vi "HEWH Check Cutout.vi"(0 "Station":string="A", 1 "Use Cutout Delay":bool, 3 "Debug":bool, 5 "Debug Events":T8, 7 "Station Data Input":T1={"Sequence #"=0.0, "Cycles"=0, "Mode Setting"="", "Flow Rate (GPM)"=0.0, "Temperature (F)"=0.0, "Reset Timer"=FALSE, "Use Temp Decline Method"=FALSE, "Terminate Condition"=enum."C1-Terminate Draw @ Gallon Mark", "Condition Value #1"=0.0, "UE"=FALSE, "LE"=FALSE, "Comp"=FALSE, "Fan"=FALSE, "Test End Time (Sec)"=0.0, "Purge Until Cutout"=FALSE, "Start Conditions"=enum."Heat Source Cutout", "Condition Value #2"=0.0, "Remove Power"=FALSE, "Time"=0.0, "Check Special Cond."=enum."SC2-Check Heat Source (On-C2/Off-C1)", "Condition#"=enum."C1", "Draw Flags"=enum."N/A", "Data Processing Delay (FHD 15sec, UEF 5 Sec)"=0.0, "Test Complete"=FALSE} {"Time" format="%<%H:%M:%S>t"}, 9 "Current (Amps)":dbl=1.0, 11 "Error In":errorcluster, 12 "Delay After Cutout (sec)":dbl=1.0, 14 "Start Draw":bool) -> (4 "Full Cutout?":bool, 15 "Error Out":errorcluster)   [LabVIEW 2016]
uses:
  Type Definitions/HEWH Power Elements.ctl
  Type Definitions/PRAT Test.ctl
  Utility/Save File/File Setup (Public)/Type Definition/Save File HEWH Heating Control Mode.ctl
  Draw Water Specific/Type Definitions/Terminate Draw Conditions.ctl
  Type Definitions/HEWH Start Conditions.ctl
  Draw Water Specific/Type Definitions/Check Special Condtions.ctl
  Draw Water Specific/Type Definitions/HEWH Special Condition Check.ctl
  Type Definitions/HEWH Draw Flag ENUM.ctl
  Utility/Type Definitions/UTILITY Notifier.ctl
  Utility/Save File/File Setup.lvlib
panel:
  out "Heat Source ON (1=ON)":bool
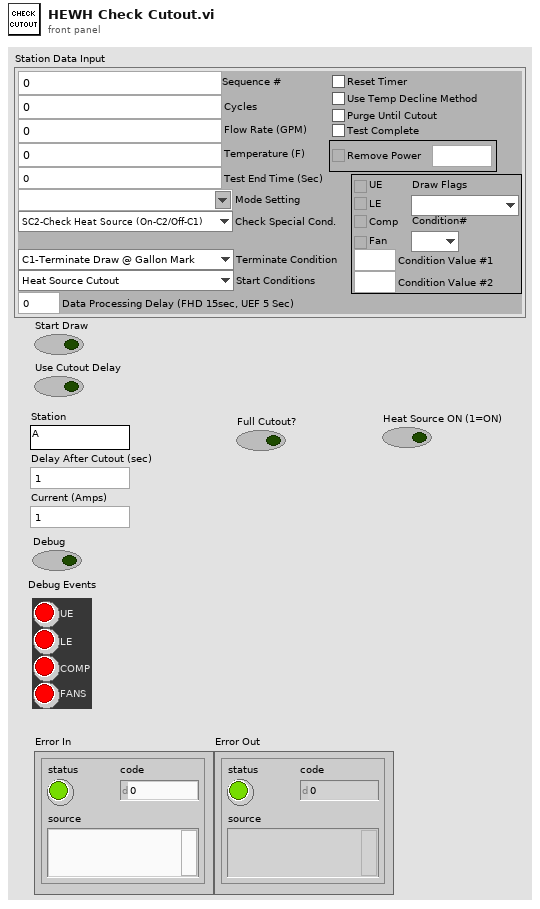
[diagram p1: front panel]
types:
  T1 = typedef "PRAT Test.ctl" = cluster{"Sequence #":dbl, "Cycles":i32, "Mode Setting":T2, "Flow Rate (GPM)":dbl, "Temperature (F)":dbl, "Reset Timer":bool, "Use Temp Decline Method":bool, "Terminate Condition":T3, "Condition Value #1":dbl, "UE":bool, "LE":bool, "Comp":bool, "Fan":bool, "Test End Time (Sec)":dbl, "Purge Until Cutout":bool, "Start Conditions":T4, "Condition Value #2":dbl, "Remove Power":bool, "Time":dbl, "Check Special Cond.":T5, "Condition#":T6, "Draw Flags":T7, "Data Processing Delay (FHD 15sec, UEF 5 Sec)":dbl, "Test Complete":bool}
  T2 = typedef "File Setup.lvlib/Save File HEWH Heating Control Mode.ctl" = string
  T3 = typedef "Terminate Draw Conditions.ctl" = enum16{"C1-Terminate Draw @ Gallon Mark", "C2-Special Last Draw (HU Test)", "C3-RTD Out <=", "C4-Mean Tank Temp <=", "C5-Decrease RTD Out (Deg F)", "C6-Time (Seconds)", "C7-Until Any Heat Source", "C8-Specific Heat Source", "C9-Do Nothing"}
  T4 = typedef "HEWH Start Conditions.ctl" = enum16{"Heat Source Cutout", "At Time (Seconds)", "Every X (Seconds)", "T2 >= X° Below Setpoint", "Seconds From Complete", "Wait for LE & Comp Cutout", "Wait for Comp Cutout", "Wait for LE Cutout", "Wait for UE Cutout"}
  T5 = typedef "Check Special Condtions.ctl" = enum16{"SC1-Do Nothing", "SC2-Check Heat Source (On-C2/Off-C1)", "SC3-Check Skip Condition", "SC4-Check Heat Source ON/Fail"}
  T6 = typedef "HEWH Special Condition Check.ctl" = enum16{"N/A", "C1", "C2", "Reset/Fail", "Skip Draw Sequence"}
  T7 = typedef "HEWH Draw Flag ENUM.ctl" = enum16{"N/A", "None(0)", "Sml(1)", "Med(2)", "SmlMed(3)", "Lrg(4)", "SmlLrg(5)", "MedLrg(6)", "SmlMedLrg(7)"}
  T8 = typedef "HEWH Power Elements.ctl" = cluster{"UE":bool, "LE":bool, "COMP":bool, "FANS":bool}
  T9 = typedef "UTILITY Notifier.ctl" = enum16{"Set", "Read", "Release Ref"}
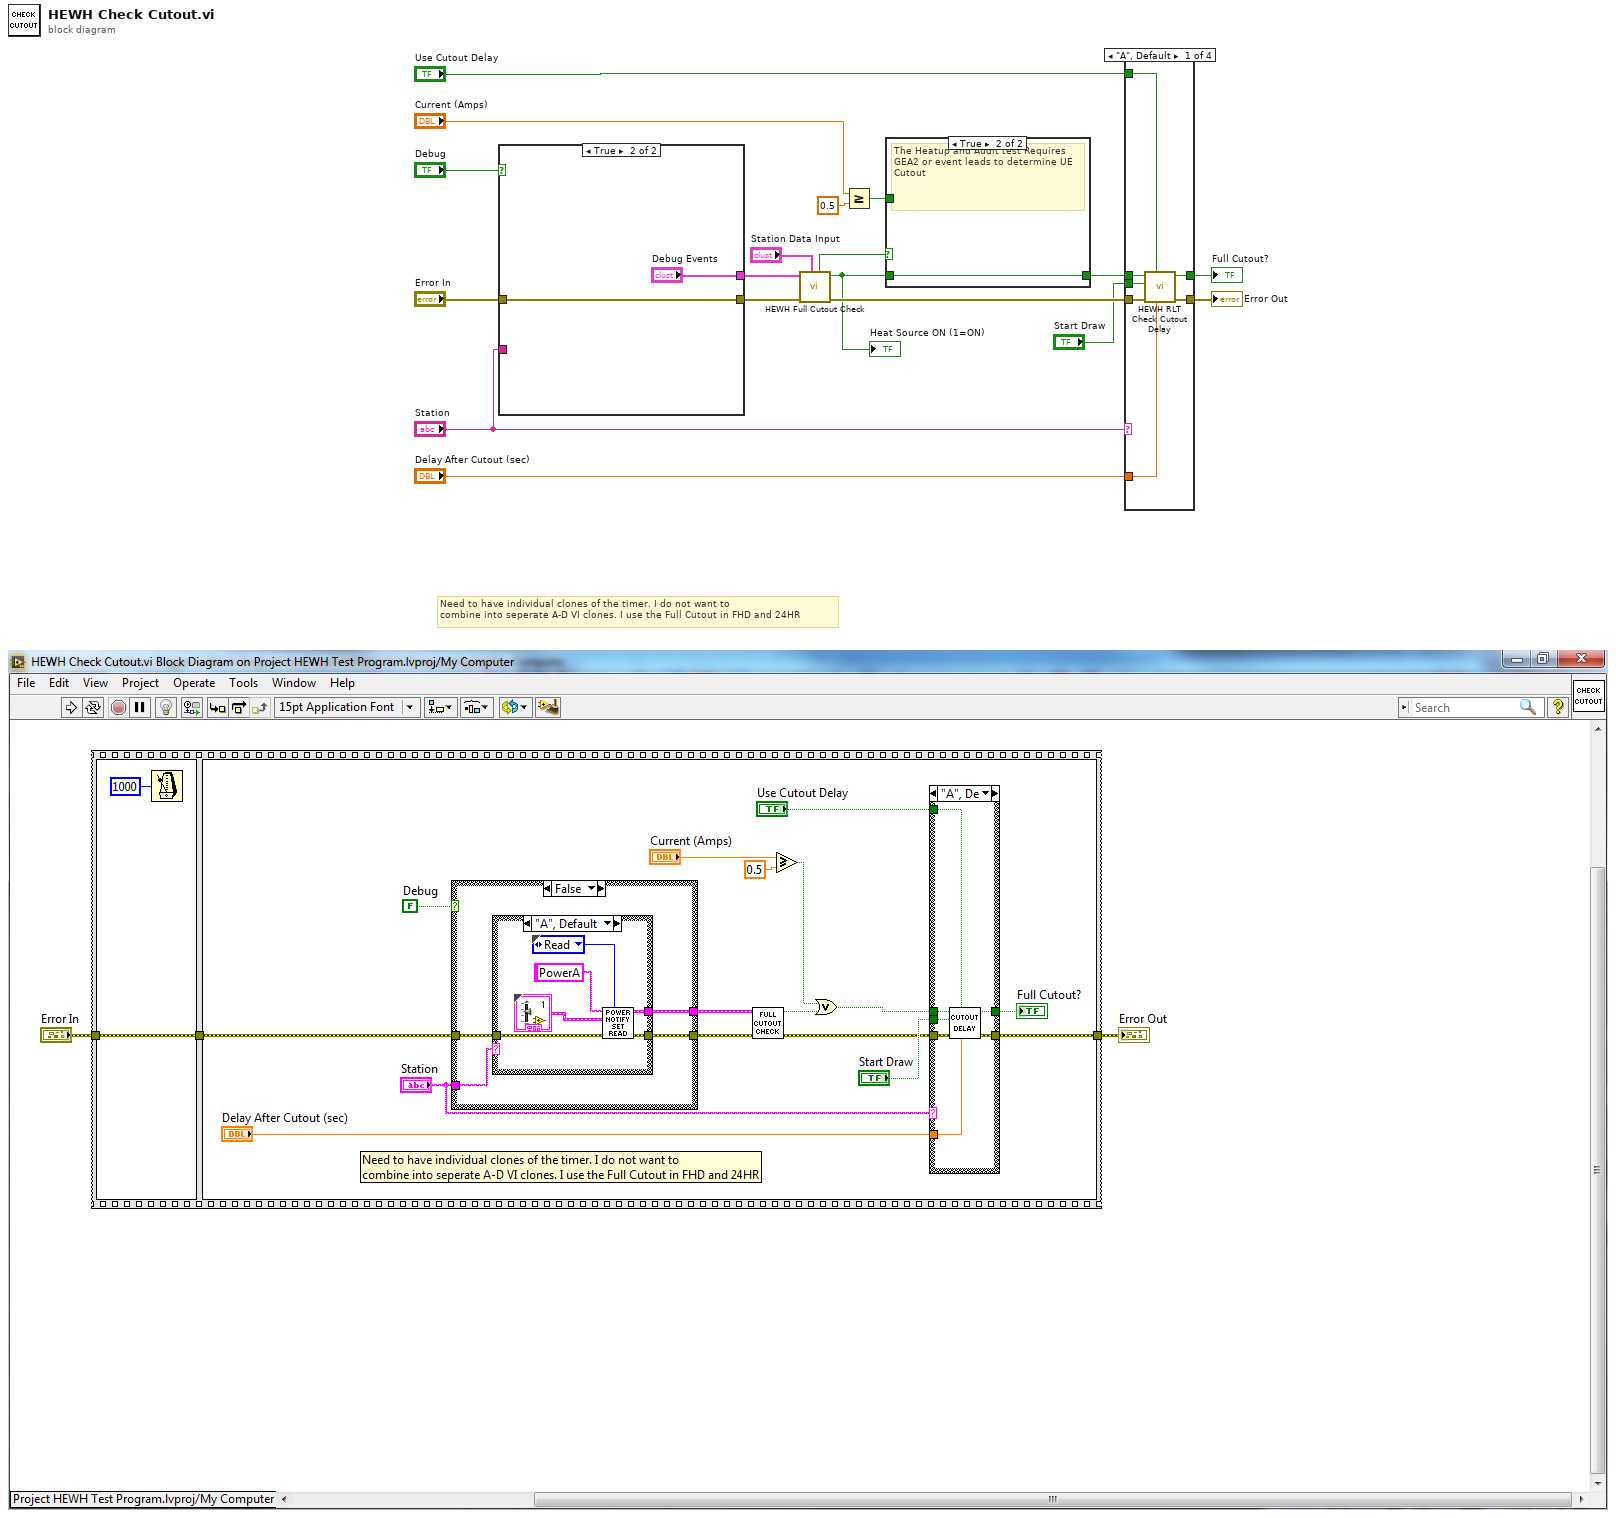
[diagram p0: block diagram]
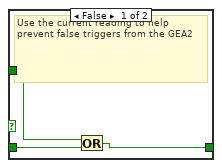
[diagram p2: hidden frame]
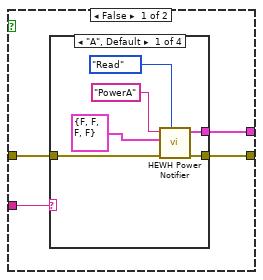
[diagram p3: hidden frame]
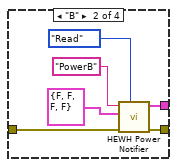
[diagram p4: hidden frame]
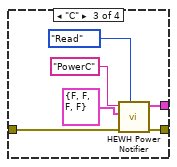
[diagram p5: hidden frame]
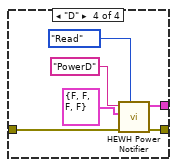
[diagram p6: hidden frame]
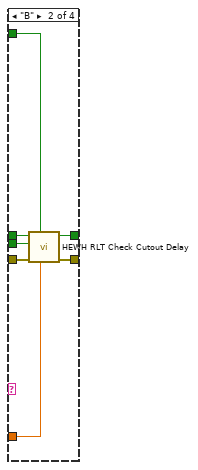
[diagram p7: hidden frame]
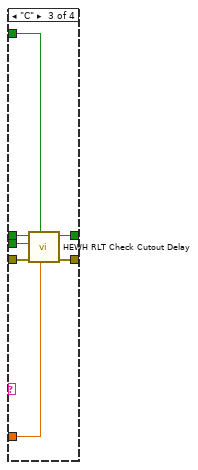
[diagram p8: hidden frame]
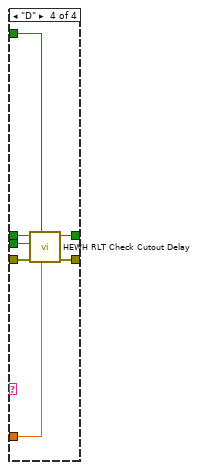
[diagram p9: hidden frame]
diagram:
  # "Need to have individual clones of the timer. I do not want to\ncombine into seperate A-D VI clones. I use the Full Cutout in FHD and 24HR"
  n1 = case shown="True" "Debug" {
    tunnel: [w22 "Debug Events"] -> w16
    tunnel: [w21 w48] -> w15
    tunnel: "Error In" -> [w20 w48]
    tunnel: "Station" -> [w19 _]
    frame False {
      n2 = case shown="\"A\", Default" w19 {
        tunnel: [w24 w30 w38 w44] -> w22
        tunnel: [w25 w31 w37 w43] -> w21
        tunnel: w20 -> [w23 w29 w35 w41]
        frame "A", Default {
          n3 = call "HEWH Power Notifier.vi"("Status"=UTILITY_Notifier."Read", "error in (no error)"=w23, "Set Status"=T8 {"UE"=FALSE, "LE"=FALSE, "COMP"=FALSE, "FANS"=FALSE}, "name (unnamed)"="PowerA") -> ("error out"=w25:errorcluster, "latest notification"=w24:T8)  [unwired: 6 in]
        }
        frame "B" {
          n4 = call "HEWH Power Notifier.vi"("Status"=UTILITY_Notifier."Read", "error in (no error)"=w29, "Set Status"=T8 {"UE"=FALSE, "LE"=FALSE, "COMP"=FALSE, "FANS"=FALSE}, "name (unnamed)"="PowerB") -> ("error out"=w31:errorcluster, "latest notification"=w30:T8)  [unwired: 6 in]
        }
        frame "C" {
          n5 = call "HEWH Power Notifier.vi"("Status"=UTILITY_Notifier."Read", "error in (no error)"=w35, "Set Status"=T8 {"UE"=FALSE, "LE"=FALSE, "COMP"=FALSE, "FANS"=FALSE}, "name (unnamed)"="PowerC") -> ("error out"=w37:errorcluster, "latest notification"=w38:T8)  [unwired: 6 in]
        }
        frame "D" {
          n6 = call "HEWH Power Notifier.vi"("Status"=UTILITY_Notifier."Read", "error in (no error)"=w41, "Set Status"=T8 {"UE"=FALSE, "LE"=FALSE, "COMP"=FALSE, "FANS"=FALSE}, "name (unnamed)"="PowerD") -> ("error out"=w43:errorcluster, "latest notification"=w44:T8)  [unwired: 6 in]
        }
      }
    }
    frame True {
    }
  }
  n7 = call "HEWH Full Cutout Check.vi"("Station Data Input"="Station Data Input", "Error In"=w15, "POWER"=w16) -> ("Error Out"=w13:errorcluster, "Heat Source ON (1=ON)"=w5:bool, "Skip Current Check"=w1:bool)  [unwired: 6 in]
  "Heat Source ON (1=ON)" <- w5
  n8 = Greater Or Equal?(x="Current (Amps)", y=0.5) -> (x >= y?=w6:bool)
  n9 = case shown="True" w1 {
    tunnel: w6 -> [w51 _]
    tunnel: w5 -> [w50 w52]
    tunnel: [w49 w52] -> w4
    frame False {
      # "Use the current reading to help\nprevent false triggers from the GEA2"
      n10 = Or(x=w51, y=w50) -> (x .or. y?=w49:bool)
    }
    frame True {
      # "The Heatup and Audit test Requires GEA2 or event leads to determine UE Cutout"
    }
  }
  n11 = case shown="\"A\", Default" "Station" {
    tunnel: [w57 w66 w71 w78] -> w7
    tunnel: "Delay After Cutout (sec)" -> [w53 w65 w68 w80]
    tunnel: w13 -> [w59 w64 w69 w75]
    tunnel: [w58 w63 w70 w79] -> w17
    tunnel: w4 -> [w55 w62 w73 w77]
    tunnel: "Use Cutout Delay" -> [w56 w61 w72 w76]
    tunnel: "Start Draw" -> [w54 w60 w67 w74]
    frame "A", Default {
      n12 = call "HEWH RLT Check Cutout Delay.vi"("Delay After Cutout (sec)"=w53, "Use Cutout Delay"=w56, "Error In"=w59, "Start Draw"=w54, "Heat Source ON (1=ON)"=w55) -> ("Error Out"=w58:errorcluster, "Full Cutout?"=w57:bool)  [unwired: 5 in]
    }
    frame "B" {
      n13 = call "HEWH RLT Check Cutout Delay.vi"("Delay After Cutout (sec)"=w65, "Use Cutout Delay"=w61, "Error In"=w64, "Start Draw"=w60, "Heat Source ON (1=ON)"=w62) -> ("Error Out"=w63:errorcluster, "Full Cutout?"=w66:bool)  [unwired: 5 in]
    }
    frame "C" {
      n14 = call "HEWH RLT Check Cutout Delay.vi"("Delay After Cutout (sec)"=w68, "Use Cutout Delay"=w72, "Error In"=w69, "Start Draw"=w67, "Heat Source ON (1=ON)"=w73) -> ("Error Out"=w70:errorcluster, "Full Cutout?"=w71:bool)  [unwired: 5 in]
    }
    frame "D" {
      n15 = call "HEWH RLT Check Cutout Delay.vi"("Delay After Cutout (sec)"=w80, "Use Cutout Delay"=w76, "Error In"=w75, "Start Draw"=w74, "Heat Source ON (1=ON)"=w77) -> ("Error Out"=w79:errorcluster, "Full Cutout?"=w78:bool)  [unwired: 5 in]
    }
  }
  "Error Out" <- w17
  "Full Cutout?" <- w7
